vi "FPH.vi"(0 "System no.":i32=1 min=1 max=4 step=1, 2 "Axes to command":string[](array[string]), 3 "All axes?":bool, 4 "Axis identifier?":bool=TRUE, 5 "error in":errorcluster) -> (19 "error out":errorcluster)   [LabVIEW 2026]
doc: "Find phase offset. See controller manual for details."
panel:
  # "Find phase offset."
  # "If all axes: use"
  # "FPH"
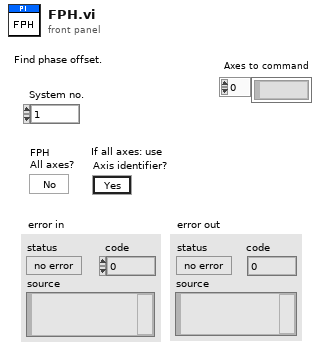
[diagram p1: front panel]
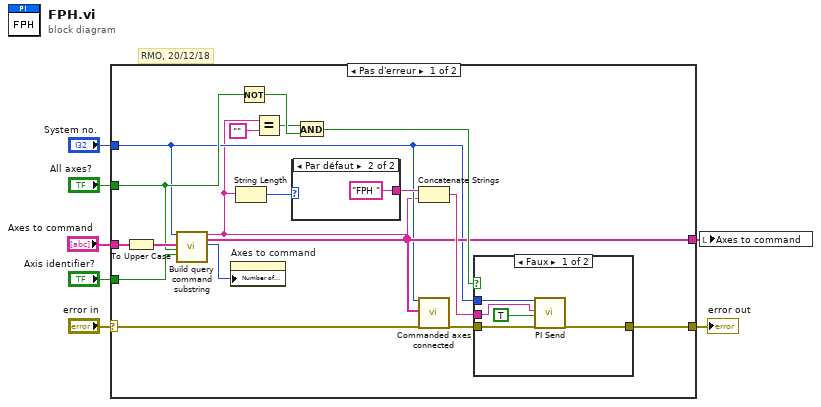
[diagram p0: block diagram]
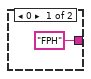
[diagram p2: hidden frame]
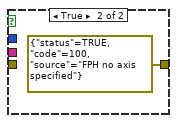
[diagram p3: hidden frame]
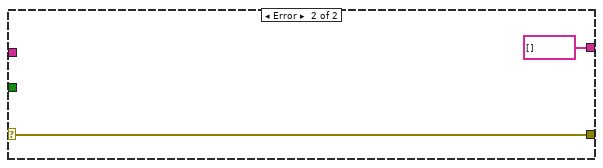
[diagram p4: hidden frame]
diagram:
  # "RMO, 20/12/18"
  n1 = case shown="Pas d'erreur" "error in" {
    selector: "error in" -> [w8 w34]
    tunnel: "System no." -> [w13 _]
    tunnel: [w25 w34] -> w6
    tunnel: "Axes to command" -> [w19 _]
    tunnel: [w17 string[] [] ("Axes to query out")] -> w3
    tunnel: "All axes?" -> [w15 _]
    tunnel: "Axis identifier?" -> [w18 _]
    frame No Error {
      n2 = To Upper Case(1:w19) -> (0:w20:string[])
      n3 = call "Build query command substring.vi"("System no."=w13, "Axes to query in"=w20, "Query\nAll axes?"=w15, "For all axes: use\nAxis identifier?"=w18) -> ("Command substring"=w10:string, "Axes to query out"=w17:string[], "Number of rows"=w12:u32)  [unwired: 1 in, 12 out]
      n4 = property on="Axes to command" class="Tabl (strict)"("Number of Rows"=w12) -> ()  [unwired: 2 in, 2 out]
      n5 = String Length(string=w10) -> (length=w9:i32)
      n6 = Not(x=w15) -> (.not. x?=w16:bool)
      n7 = Equal?(x=w10, y="") -> (x = y?=w14:bool)
      n8 = case shown="Par défaut" w9 {
        tunnel: ["FPH" ("string") "FPH " ("string")] -> w21
        frame 0 {
        }
        frame Default {
        }
      }
      n9 = And(x=w14, y=w16) -> (x .and. y?=w22:bool)
      n10 = Concatenate Strings(w21, w10) -> (w23:string)
      n11 = call "Commanded axes connected.vi"("System no."=w13, "Commanded axes"=w17, "error in"=w8) -> ("error out"=w24:errorcluster)  [unwired: 16 out]
      n12 = case shown="Faux" w22 {
        tunnel: [w31 errorcluster {"status"=TRUE, "code"=100, "source"="FPH no axis specified"} ("error out")] -> w25
        tunnel: w24 -> [w30 _]
        tunnel: w23 -> [w28 _]
        tunnel: w13 -> [w29 _]
        frame False {
          n13 = call "PI Send.vi"("System no."=w29, "String to send"=w28, "Attach termination char.?"=TRUE ("Attach Linefeed?"), "error in"=w30) -> ("error out"=w31:errorcluster)  [unwired: 2 in, 13 out]
        }
        frame True {
        }
      }
    }
    frame Error {
    }
  }
  "error out" <- w6
  n14 = local write "Axes to command"(w3) -> ()
